vi "内存中所有的VI属性.vi"() -> ()   [LabVIEW 2011]
panel:
  out "Application:All VIs In Memory":string[](array[string])
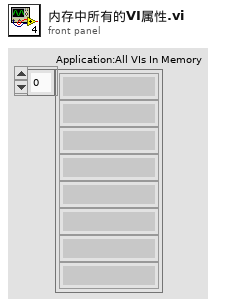
[diagram p1: front panel]
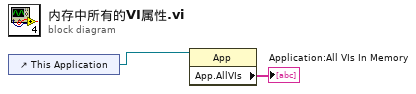
[diagram p0: block diagram]
diagram:
  n1 = control-ref of="This Application"() -> (w2:refnum<vi>)
  n2 = property class="App"(reference=w2) -> ("App.AllVIs"=→"Application:All VIs In Memory":string[])  [unwired: 1 in, 2 out]
